vi "221013_CreateRInOhm.vi"(2 "error in (no error)":errorcluster, 3 "Lower Bound":i64=90, 4 "Upper Bound":i64=110, 5 "Number of Values":i32=1) -> (0 "error out":errorcluster, 1 "Array Out":i64[](array[numeric]))   [LabVIEW 2022 SP3]
doc: "Erzeugt die Anzahl an Zufallszahlen zwischen den Grenzwerten (Upper Bound, Lower Bound)"
uses:
  <vilib>/numeric/Random Number (Range) I64.vi
  <vilib>/numeric/sub_Random U32.vi
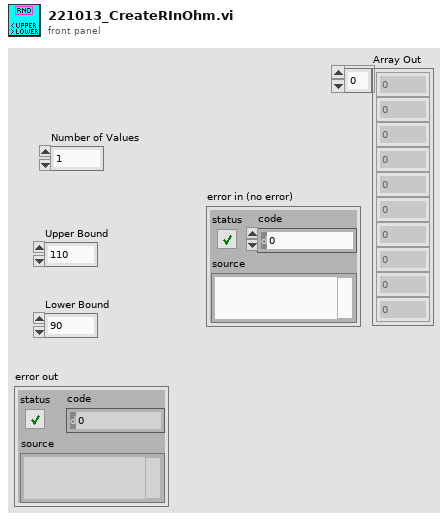
[diagram p1: front panel]
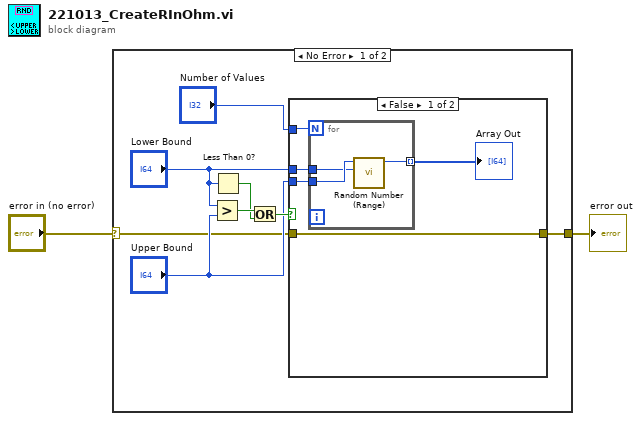
[diagram p0: block diagram]
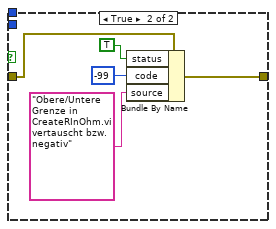
[diagram p2: hidden frame]
diagram:
  n1 = case shown="No Error" "error in (no error)" {
    selector: "error in (no error)" -> [w5 w24]
    tunnel: [w4 w24] -> w1
    frame No Error {
      n2 = Greater?(x="Lower Bound", y="Upper Bound") -> (0:w10:bool)
      n3 = Less Than 0?(x="Lower Bound") -> (x < 0?=w9:bool)
      n4 = Or(x=w10, y=w9) -> (x .or. y?=w8:bool)
      n5 = case shown="False" w8 {
        tunnel: "Number of Values" -> [w15 _]
        tunnel: "Upper Bound" -> [w14 _]
        tunnel: "Lower Bound" -> [w13 _]
        tunnel: w5 -> [w11 w23]
        tunnel: [w11 w22] -> w4
        frame False {
          n6 = for {
            N: w15 -> [_]
            tunnel: w14 -> [w18]
            tunnel: w13 -> [w17]
            tunnel: [w16] -> w12 mode=indexing
            n7 = call-poly <vilib>:"Random Number (Range).vi"("lower bound (-100)"=w17, "upper bound (100)"=w18) -> ("number"=w16:i64)  [unwired: 9 in]
          }
          "Array Out" <- w12
        }
        frame True {
          n8 = Bundle By Name(cluster=w23, "status"=TRUE, "code"=-99, "source"="Obere/Untere Grenze in CreateRInOhm.vi vertauscht bzw. negativ") -> (w22:errorcluster)
        }
      }
    }
    frame Error {
    }
  }
  "error out" <- w1
